vi "HEWH FHD Modify for UE LE Draw.vi"(6 "Electric Water Heater (Lowboy)?":bool, 8 "Error In":errorcluster, 9 "Gas Water Heater?":bool, 10 "Electric Water Heater (40/50 gallon)?":bool, 11 "1st HR Test in":T1[](array[typedef])=[{"Sequence #"=1.0, "Cycles"=1, "Mode Setting"="", "Flow Rate (GPM)"=3.0, "Temperature (F)"=58.0, "Reset Timer"=FALSE, "Use Temp Decline Method"=FALSE, "Terminate Condition"=enum."C7-Until Any Heat Source", "Condition Value #1"=0.0, "UE"=TRUE, "LE"=TRUE, "Comp"=FALSE, "Fan"=FALSE, "Test End Time (Sec)"=0.0, "Purge Until Cutout"=FALSE, "Start Conditions"=enum."Heat Source Cutout", "Condition Value #2"=180.0, "Remove Power"=TRUE, "Time"=3600.0, "Check Special Cond."=enum."SC1-Do Nothing", "Condition#"=enum."N/A", "Draw Flags"=enum."N/A", "Data Processing Delay (FHD 15sec, UEF 5 Sec)"=15.0, "Test Complete"=FALSE, "User Setpoint"=0.0, "Tank Setpoint"=0.0}, {"Sequence #"=2.0, "Cycles"=1, "Mode Setting"="", "Flow Rate (GPM)"=3.0, "Temperature (F)"=58.0, "Reset Timer"=TRUE, "Use Temp Decline Method"=TRUE, "Terminate Condition"=enum."C5-Decrease RTD Out (Deg F)", "Condition Value #1"=0.0, "UE"=TRUE, "LE"=TRUE, "Comp"=FALSE, "Fan"=FALSE, "Test End Time (Sec)"=0.0, "Purge Until Cutout"=FALSE, "Start Conditions"=enum."Heat Source Cutout", "Condition Value #2"=180.0, "Remove Power"=TRUE, "Time"=3600.0, "Check Special Cond."=enum."SC1-Do Nothing", "Condition#"=enum."N/A", "Draw Flags"=enum."N/A", "Data Processing Delay (FHD 15sec, UEF 5 Sec)"=15.0, "Test Complete"=FALSE, "User Setpoint"=0.0, "Tank Setpoint"=0.0}, {"Sequence #"=3.0, "Cycles"=5, "Mode Setting"="", "Flow Rate (GPM)"=3.0, "Temperature (F)"=58.0, "Reset Timer"=FALSE, "Use Temp Decline Method"=FALSE, "Terminate Condition"=enum."C5-Decrease RTD Out (Deg F)", "Condition Value #1"=0.0, "UE"=TRUE, "LE"=TRUE, "Comp"=FALSE, "Fan"=FALSE, "Test End Time (Sec)"=0.0, "Purge Until Cutout"=TRUE, "Start Conditions"=enum."T2 >= X° Below Setpoint", "Condition Value #2"=180.0, "Remove Power"=TRUE, "Time"=3600.0, "Check Special Cond."=enum."SC1-Do Nothing", "Condition#"=enum."N/A", "Draw Flags"=enum."N/A", "Data Processing Delay (FHD 15sec, UEF 5 Sec)"=15.0, "Test Complete"=FALSE, "User Setpoint"=0.0, "Tank Setpoint"=0.0}, {"Sequence #"=4.0, "Cycles"=1, "Mode Setting"="", "Flow Rate (GPM)"=3.0, "Temperature (F)"=58.0, "Reset Timer"=FALSE, "Use Temp Decline Method"=FALSE, "Terminate Condition"=enum."C2-Special Last Draw (HU Test)", "Condition Value #1"=0.0, "UE"=TRUE, "LE"=TRUE, "Comp"=FALSE, "Fan"=FALSE, "Test End Time (Sec)"=3600.0, "Purge Until Cutout"=TRUE, "Start Conditions"=enum."Seconds From Complete", "Condition Value #2"=180.0, "Remove Power"=TRUE, "Time"=3600.0, "Check Special Cond."=enum."SC1-Do Nothing", "Condition#"=enum."N/A", "Draw Flags"=enum."N/A", "Data Processing Delay (FHD 15sec, UEF 5 Sec)"=15.0, "Test Complete"=FALSE, "User Setpoint"=0.0, "Tank Setpoint"=0.0}] {"Time" format="%<%H:%M:%S>t"}) -> (0 "Error Out":errorcluster, 3 "1st HR Test out":T1[](array[typedef]) {"Time" format="%<%H:%M:%S>t"})   [LabVIEW 2019]
uses:
  Type Definitions/PRAT Test.ctl
  Utility/Save File/File Setup (Public)/Type Definition/Save File HEWH Heating Control Mode.ctl
  Draw Water Specific/Type Definitions/Terminate Draw Conditions.ctl
  Type Definitions/HEWH Start Conditions.ctl
  Draw Water Specific/Type Definitions/Check Special Condtions.ctl
  Draw Water Specific/Type Definitions/HEWH Special Condition Check.ctl
  Type Definitions/HEWH Draw Flag ENUM.ctl
  Utility/Save File/File Setup.lvlib
panel:
  # "Uncheck LE if UE actuates during the FHD\nCheck LE if UE DOES NOT actuate during FHD"
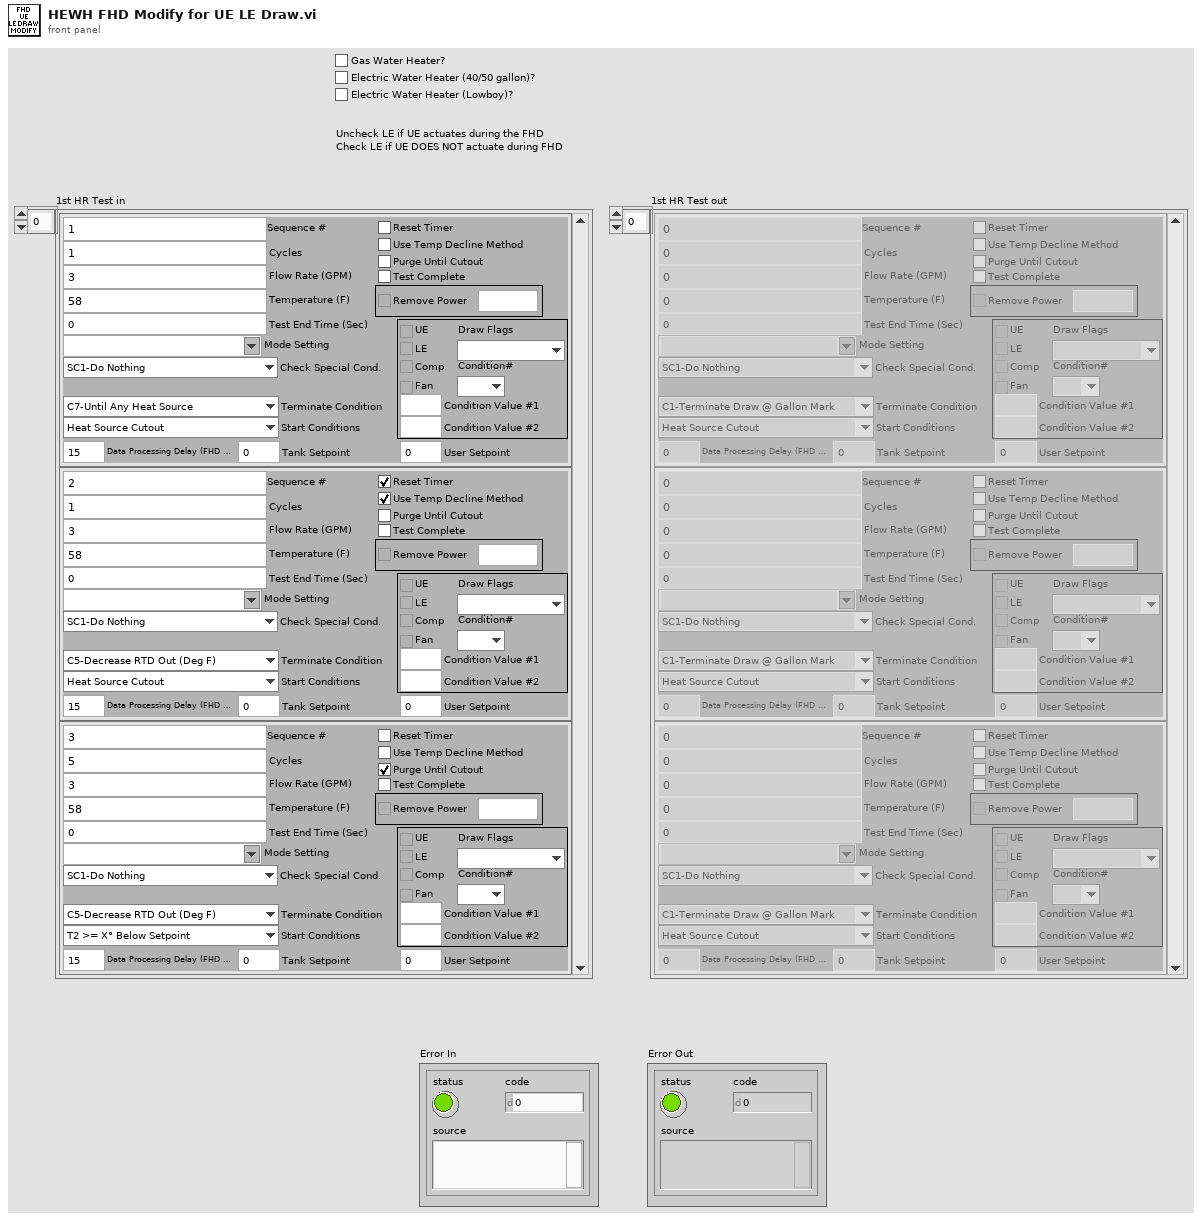
[diagram p1: front panel]
types:
  T1 = typedef "PRAT Test.ctl" = cluster{"Sequence #":dbl, "Cycles":i32, "Mode Setting":T2, "Flow Rate (GPM)":dbl, "Temperature (F)":dbl, "Reset Timer":bool, "Use Temp Decline Method":bool, "Terminate Condition":T3, "Condition Value #1":dbl, "UE":bool, "LE":bool, "Comp":bool, "Fan":bool, "Test End Time (Sec)":dbl, "Purge Until Cutout":bool, "Start Conditions":T4, "Condition Value #2":dbl, "Remove Power":bool, "Time":dbl, "Check Special Cond.":T5, "Condition#":T6, "Draw Flags":T7, "Data Processing Delay (FHD 15sec, UEF 5 Sec)":dbl, "Test Complete":bool, "User Setpoint":dbl, "Tank Setpoint":dbl}
  T2 = typedef "File Setup.lvlib/Save File HEWH Heating Control Mode.ctl" = string
  T3 = typedef "Terminate Draw Conditions.ctl" = enum16{"C1-Terminate Draw @ Gallon Mark", "C2-Special Last Draw (HU Test)", "C3-RTD Out <=", "C4-Mean Tank Temp <=", "C5-Decrease RTD Out (Deg F)", "C6-Time (Seconds)", "C7-Until Any Heat Source", "C8-Specific Heat Source", "C9-Do Nothing", "C10-Inlet Outlet RTD Temp Delta"}
  T4 = typedef "HEWH Start Conditions.ctl" = enum16{"Heat Source Cutout", "At Time (Seconds)", "Every X (Seconds)", "T2 >= X° Below Setpoint", "Seconds From Complete", "Wait for LE & Comp Cutout", "Wait for Comp Cutout", "Wait for LE Cutout", "Wait for UE Cutout", "Start Immediately"}
  T5 = typedef "Check Special Condtions.ctl" = enum16{"SC1-Do Nothing", "SC2-Check Heat Source (On-C2/Off-C1)", "SC3-Check Skip Condition", "SC4-Check Heat Source ON/Fail", "SC5-Keep Draw Valves Open", "SC6-Skip Purge"}
  T6 = typedef "HEWH Special Condition Check.ctl" = enum16{"N/A", "C1", "C2", "Reset/Fail", "Skip Draw Sequence"}
  T7 = typedef "HEWH Draw Flag ENUM.ctl" = enum16{"N/A", "None(0)", "Sml(1)", "Med(2)", "SmlMed(3)", "Lrg(4)", "SmlLrg(5)", "MedLrg(6)", "SmlMedLrg(7)"}
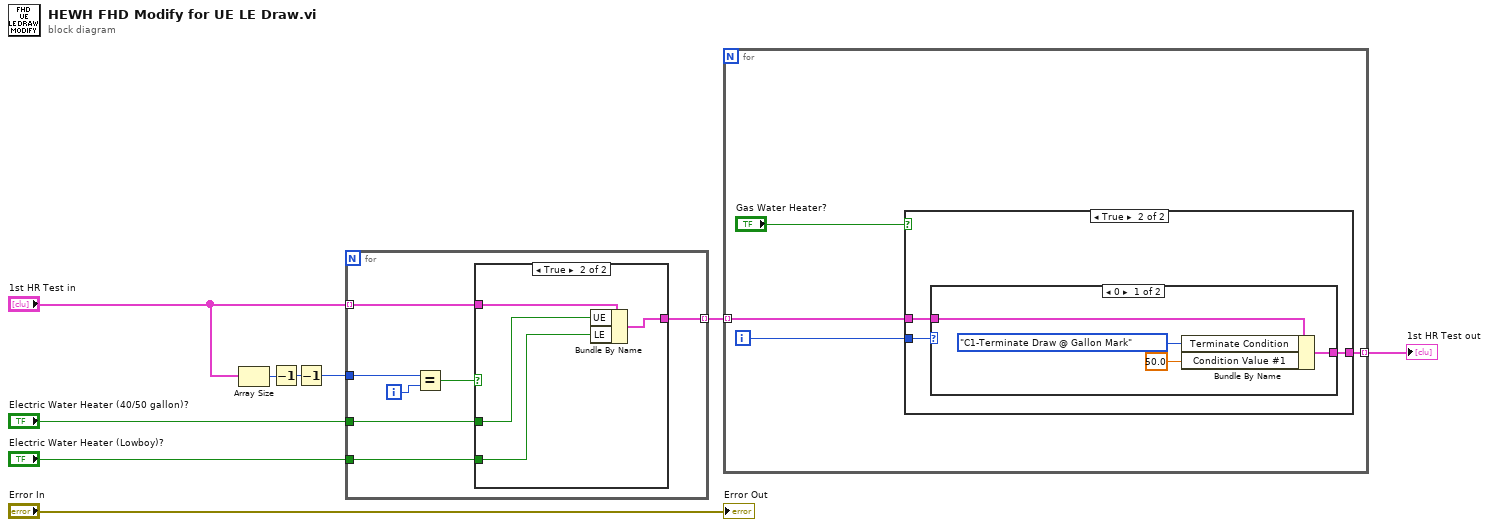
[diagram p0: block diagram]
diagram:
  n1 = Array Size(array="1st HR Test in") -> (size(s)=w9:i32)
  n2 = Decrement(x=w9) -> (x-1=w8:i32)
  n3 = Decrement(x=w8) -> (x-1=w6:i32)
  n4 = for {
    tunnel: "1st HR Test in" -> [w13] mode=indexing
    tunnel: w6 -> [w15]
    tunnel: "Electric Water Heater (40/50 gallon)?" -> [w12]
    tunnel: [w11] -> w4 mode=indexing
    tunnel: "Electric Water Heater (Lowboy)?" -> [w10]
    i -> [w16]
    n5 = Equal?(x=w15, y=w16) -> (x = y?=w14:bool)
    n6 = case shown="True" w14 {
      tunnel: w13 -> [w17 w21]
      tunnel: w12 -> [_ w19]
      tunnel: [w17 w20] -> w11
      tunnel: w10 -> [_ w18]
      frame False {
      }
      frame True {
        n7 = Bundle By Name(cluster=w21, "UE"=w19, "LE"=w18) -> (w20:T1)
      }
    }
  }
  n8 = for {
    tunnel: w4 -> [w25] mode=indexing
    tunnel: [w23] -> w3 mode=indexing
    i -> [w24]
    n9 = case shown="True" "Gas Water Heater?" {
      tunnel: w25 -> [w26 w29]
      tunnel: w24 -> [_ w28]
      tunnel: [w26 w27] -> w23
      frame False {
      }
      frame True {
        n10 = case shown="0" w28 {
          tunnel: w29 -> [w33 w34]
          tunnel: [w32 w34] -> w27
          frame 0 {
            n11 = Bundle By Name(cluster=w33, "Terminate Condition"=Terminate_Draw_Conditions."C1-Terminate Draw @ Gallon Mark", "Condition Value #1"=50.0) -> (w32:T1)
          }
          frame 1, Default {
          }
        }
      }
    }
  }
  "1st HR Test out" <- w3
  "Error Out" <- "Error In"
